vi "Mapping.vi"(0 "DBL Input":dbl, 5 "DBL Input 2":dbl, 7 "DBL Input 3":dbl, 9 "DBL Input 4":dbl, 11 "DBL Input 5":dbl) -> (4 "Poker output":dbl, 6 "Poker output 2":dbl, 8 "Poker output 3":dbl, 10 "Poker output 4":dbl, 15 "Poker output 5":dbl)   [LabVIEW 2014]
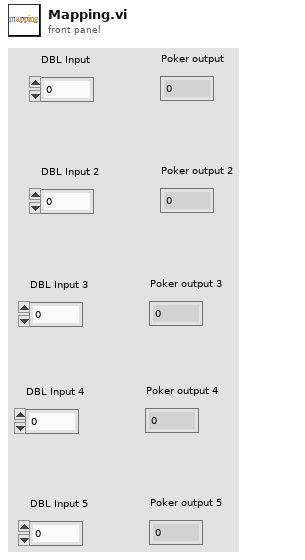
[diagram p1: front panel]
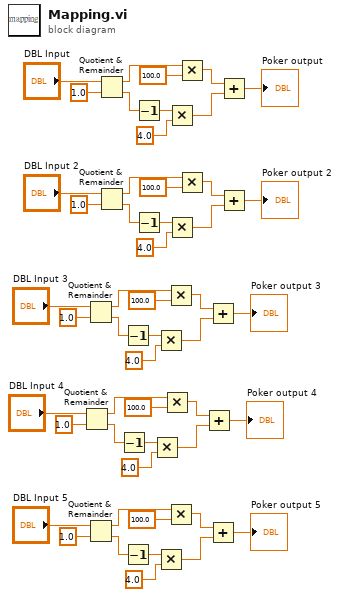
[diagram p0: block diagram]
diagram:
  n1 = Quotient & Remainder(x="DBL Input 4", y=1.0) -> (x-y*floor(x/y)=w14:dbl, floor(x/y)=w13:dbl)
  n2 = Quotient & Remainder(x="DBL Input 3", y=1.0) -> (x-y*floor(x/y)=w27:dbl, floor(x/y)=w28:dbl)
  n3 = Quotient & Remainder(x="DBL Input 5", y=1.0) -> (x-y*floor(x/y)=w7:dbl, floor(x/y)=w8:dbl)
  n4 = Quotient & Remainder(x="DBL Input", y=1.0) -> (x-y*floor(x/y)=w47:dbl, floor(x/y)=w48:dbl)
  n5 = Quotient & Remainder(x="DBL Input 2", y=1.0) -> (x-y*floor(x/y)=w34:dbl, floor(x/y)=w33:dbl)
  n6 = Decrement(x=w13) -> (x-1=w18:dbl)
  n7 = Decrement(x=w28) -> (x-1=w23:dbl)
  n8 = Decrement(x=w8) -> (x-1=w3:dbl)
  n9 = Decrement(x=w48) -> (x-1=w43:dbl)
  n10 = Decrement(x=w33) -> (x-1=w38:dbl)
  n11 = Multiply(x=w18, y=4.0) -> (x*y=w20:dbl)
  n12 = Multiply(x=w23, y=4.0) -> (x*y=w21:dbl)
  n13 = Multiply(x=w3, y=4.0) -> (x*y=w1:dbl)
  n14 = Multiply(x=w14, y=100.0) -> (x*y=w16:dbl)
  n15 = Multiply(x=w27, y=100.0) -> (x*y=w25:dbl)
  n16 = Multiply(x=w7, y=100.0) -> (x*y=w5:dbl)
  n17 = Multiply(x=w43, y=4.0) -> (x*y=w41:dbl)
  n18 = Multiply(x=w38, y=4.0) -> (x*y=w40:dbl)
  n19 = Multiply(x=w47, y=100.0) -> (x*y=w45:dbl)
  n20 = Multiply(x=w34, y=100.0) -> (x*y=w36:dbl)
  n21 = Add(x=w16, y=w20) -> (x+y=→"Poker output 4":dbl)
  n22 = Add(x=w25, y=w21) -> (x+y=→"Poker output 3":dbl)
  n23 = Add(x=w5, y=w1) -> (x+y=→"Poker output 5":dbl)
  n24 = Add(x=w45, y=w41) -> (x+y=→"Poker output":dbl)
  n25 = Add(x=w36, y=w40) -> (x+y=→"Poker output 2":dbl)
